vi "Mark Passoffs.vi"(8 "error in":errorcluster, 11 "Array in":T1[](array[typedef]) {"Creation Date" format="%<%x>T"; "Last Updated" format="%<%x>T"}) -> (0 "error out":errorcluster, 3 "Array out":T1[](array[typedef]) {"Creation Date" format="%<%x>T"; "Last Updated" format="%<%x>T"})   [LabVIEW 2018]
uses:
  Type Defs/SR Cluster.ctl
  Type Defs/SR Status.ctl
  Type Defs/FGV States.ctl
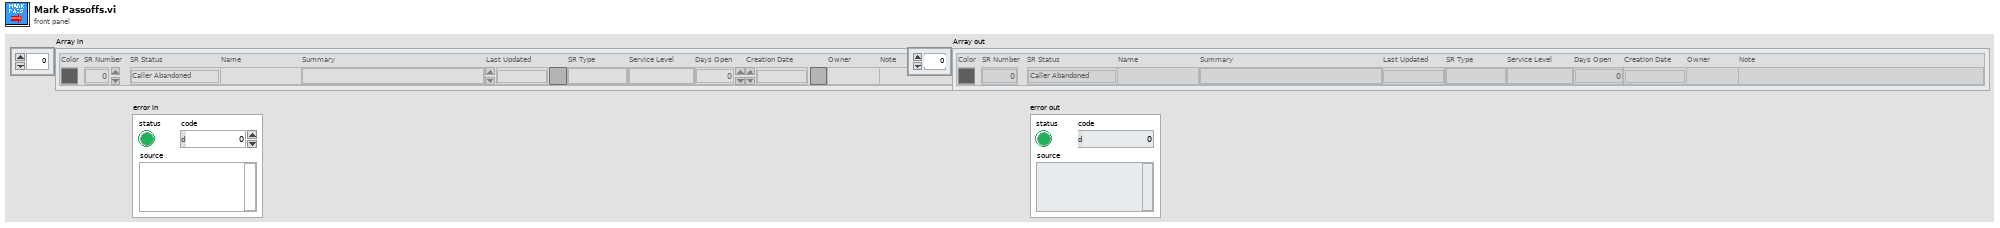
[diagram p1: front panel]
types:
  T1 = typedef "SR Cluster.ctl" = cluster{"Color":u32, "SR Number":i32, "SR Status":T2, "Name":string, "Summary":string, "Last Updated":timestamp, "SR Type":string, "Service Level":string, "Days Open":dbl, "Creation Date":timestamp, "Owner":string, "Note":string}
  T2 = typedef "SR Status.ctl" = enum16{"Caller Abandoned", "Created in Error", "Expired", "Forum Resolved AE", "Forum Resolved Customer", "IN WORK", "IN WORK Collab with AES", "IN WORK Collab with PSE", "IN WORK Collab with SE", "IN WORK Customer Added Note", "IN WORK Escalation", "IN WORK Wait on Customer", "Open", "Potentially Resolved", "Presumed Resolved", "RMA Approved for Return", "RMA Closed", "RMA Closed - DOA", "RMA In Progress", "RMA Open", "RMA Waiting on Customer", "Resolved", "Passed Off"}
  T3 = typedef "FGV States.ctl" = enum16{"Initialize", "Merge", "Write", "Remove", "Read", "Clear"}
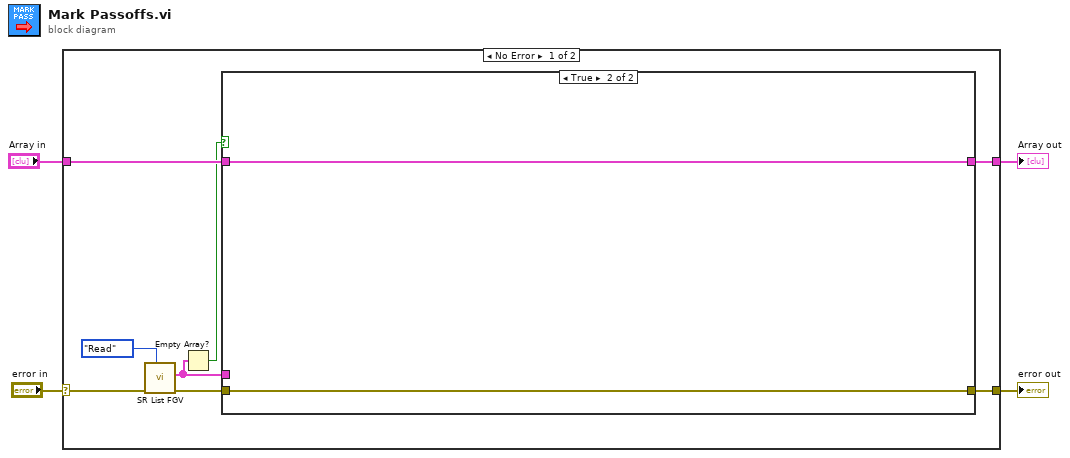
[diagram p0: block diagram]
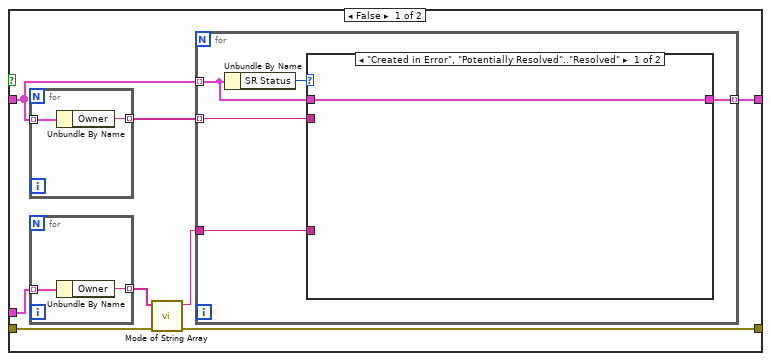
[diagram p2: hidden frame]
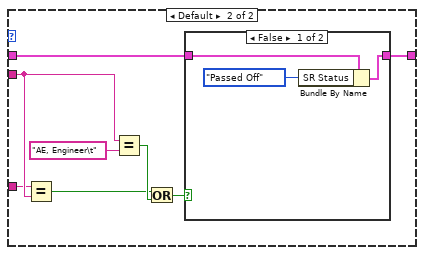
[diagram p3: hidden frame]
diagram:
  n1 = case shown="No Error" "error in" {
    selector: "error in" -> [w10 w46]
    tunnel: "Array in" -> [w12 w45]
    tunnel: [w11 w45] -> w3
    tunnel: [w9 w46] -> w2
    frame No Error {
      n2 = call "SR List FGV.vi"("Operation"=FGV_States."Read", "Error In"=w10) -> ("Error Out"=w8:errorcluster, "list out"=w5:T1[])  [unwired: 8 in]
      n3 = Empty Array?(array=w5) -> (empty?=w6:bool)
      n4 = case shown="True" w6 {
        tunnel: w12 -> [w19 w44]
        tunnel: [w18 w44] -> w11
        tunnel: [w16 w43] -> w9
        tunnel: w5 -> [w15 _]
        tunnel: w8 -> [w13 w43]
        frame False {
          n5 = for {
            tunnel: w19 -> [w42] mode=indexing
            tunnel: [w41] -> w20 mode=indexing
            n6 = Unbundle By Name(w42) -> ("Owner"=w41:string)
          }
          n7 = for {
            tunnel: w15 -> [w22] mode=indexing
            tunnel: [w21] -> w14 mode=indexing
            n8 = Unbundle By Name(w22) -> ("Owner"=w21:string)
          }
          n9 = call "Mode of String Array.vi"("error in"=w13, "Input Elements"=w14) -> ("error out"=w16:errorcluster, "most frequent"=w17:string)  [unwired: 7 in, 1 out]
          n10 = for {
            tunnel: w20 -> [w27] mode=indexing
            tunnel: w19 -> [w24] mode=indexing
            tunnel: [w25] -> w18 mode=indexing
            tunnel: w17 -> [w26]
            n11 = Unbundle By Name(w24) -> ("SR Status"=w23:T2)
            n12 = case shown="\"Created in Error\", \"Potentially Resolved\"..\"Resolved\"" w23 {
              tunnel: w27 -> [_ w32]
              tunnel: w26 -> [_ w31]
              tunnel: w24 -> [w28 w29]
              tunnel: [w28 w30] -> w25
              frame "Created in Error", "Potentially Resolved".."Resolved" {
              }
              frame Default {
                n13 = Equal?(x=w31, y=w32) -> (x = y?=w34:bool)
                n14 = Equal?(x=w32, y="AE, Engineer\t" ("t")) -> (x = y?=w35:bool)
                n15 = Or(x=w34, y=w35) -> (x .or. y?=w36:bool)
                n16 = case shown="False" w36 {
                  tunnel: [w38 w40] -> w30
                  tunnel: w29 -> [w39 w40]
                  frame False {
                    n17 = Bundle By Name(cluster=w39, "SR Status"=SR_Status."Passed Off") -> (w38:T1)
                  }
                  frame True {
                  }
                }
              }
            }
          }
        }
        frame True {
        }
      }
    }
    frame Error {
    }
  }
  "error out" <- w2
  "Array out" <- w3
